vi "Get Class Data.vi"(7 "Object":refnum<class>, 8 "error in (no error)":errorcluster, 10 "Class default data":variant[](array[variant]), 11 "CConfig Variant Accessor in":refnum<class "CConfig Variant Accessor.lvclass">) -> (0 "error out":errorcluster, 2 "Class data":variant[](array[variant]), 3 "CConfig Variant Accessor out":refnum<class "CConfig Variant Accessor.lvclass">, 5 "Object (dup)":refnum<class>)   [LabVIEW 2013, in "CConfig Variant Accessor.lvclass"]
doc: "Copyright 2018, Carya Automatisering, Wiebe Walstra."
uses:
  CConfig Variant Accessor.lvclass
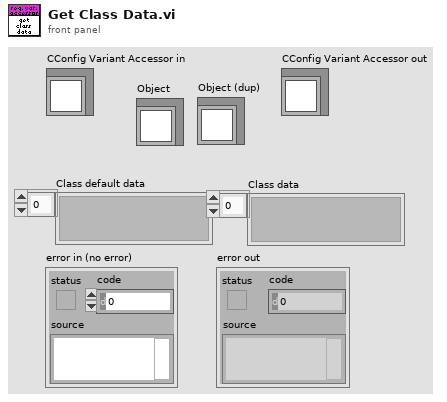
[diagram p1: front panel]
types:
  T1 = cluster{"levels":i32, "h.size":u8, "name size":u8}
  T2 = cluster{"v.major":u16, "v.minor":u16, "v.fix":u16, "v.build":u16}
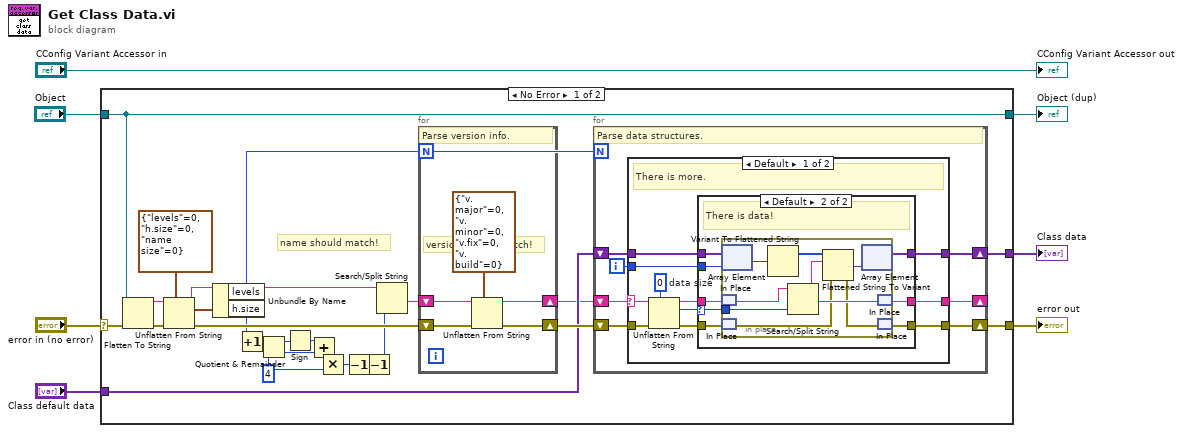
[diagram p0: block diagram]
diagram:
  n1 = case shown="No Error" "error in (no error)" {
    selector: "error in (no error)" -> [w24 w81]
    tunnel: [w23 w81] -> w6
    tunnel: "Object" -> [w22 w80]
    tunnel: [w22 w80] -> w3
    tunnel: "Class default data" -> [w21 w79]
    tunnel: [w20 w79] -> w1
    frame No Error {
      w19 = u8 4 ("y")
      # "name should match!"
      n2 = Flatten To String(anything=w22, error in (no error)=w24) -> (data string=w25:string, error out=w26:errorcluster)  [unwired: 2 in, 1 out]
      n3 = Unflatten From String(type=T1 {"levels"=0, "h.size"=0, "name size"=0}, binary string=w25, error in (no error)=w26) -> (rest of the binary string=w31:string, value=w30:T1, error out=w28:errorcluster)  [unwired: 2 in]
      n4 = Unbundle By Name(w30) -> ("levels"=w29:i32, "h.size"=w11:u8)
      n5 = Increment(x=w11) -> (x+1=w10:u8)
      n6 = Quotient & Remainder(x=w10, y=w19) -> (x-y*floor(x/y)=w16:u8, floor(x/y)=w18:u8)
      n7 = Sign(1:w16) -> (0:w15:u8)
      n8 = Add(x=w15, y=w18) -> (x+y=w17:u8)
      n9 = Multiply(x=w17, y=w19) -> (x*y=w14:u8)
      n10 = Decrement(x=w14) -> (x-1=w9:u8)
      n11 = Decrement(x=w9) -> (x-1=w8:u8)
      n12 = Search/Split String(string=w31, offset (0)=w8) -> (match + rest of string=w12:string)  [unwired: 1 in, 2 out]
      n13 = for {
        N: w29 -> [_]
        shift-right: [w33] -> w27
        shift-left: w28 -> [w36]
        shift-right: [w34] -> w13
        shift-left: w12 -> [w35]
        # "version should match!"
        # "Parse version info."
        n14 = Unflatten From String(type=T2 {"v.major"=0, "v.minor"=0, "v.fix"=0, "v.build"=0}, binary string=w35, error in (no error)=w36) -> (rest of the binary string=w34:string, error out=w33:errorcluster)  [unwired: 2 in, 1 out]
      }
      n15 = for {
        N: w29 -> [_]
        shift-right: [w43] -> w23
        shift-left: w27 -> [w42]
        shift-right: [w44] -> _
        shift-left: w13 -> [w41]
        shift-right: [w39] -> w20
        shift-left: w21 -> [w40]
        i -> [w38]
        # "Parse data structures."
        n16 = case shown="Default" w41 {
          selector: w41 -> [w50 w77]
          tunnel: w42 -> [w55 w78]
          tunnel: [w51 w77] -> w44
          tunnel: [w47 w78] -> w43
          tunnel: w40 -> [w49 w76]
          tunnel: [w48 w76] -> w39
          tunnel: w38 -> [w45 _]
          frame Default {
            w54 = 0  # data size
            # "There is more."
            n17 = Unflatten From String(type=w54, binary string=w50, error in (no error)=w55) -> (rest of the binary string=w52:string, value=w53:i32, error out=w46:errorcluster)  [unwired: 2 in]
            n18 = case shown="Default" w53 {
              selector: w53 -> [_ w66]
              tunnel: w52 -> [w58 w62]
              tunnel: [w58 w61] -> w51
              tunnel: w49 -> [w57 w65]
              tunnel: [w57 w64] -> w48
              tunnel: [w56 w59] -> w47
              tunnel: w46 -> [w56 w60]
              tunnel: w45 -> [_ w63]
              frame 0 {
                # "Data size is 0. Must be default."
              }
              frame Default {
                # "There is data!"
                n19 = in-place {
                  in-place-border: w66 -> [w75]
                  n20 = in-place-array #1(w65, w63) -> (w72:variant)
                  n21 = in-place-match #2(w62) -> (w70:string)
                  n22 = in-place-match #3(w60) -> (w68:errorcluster)
                  n23 = Variant To Flattened String(Variant=w72) -> (1:w73:i16[])  [unwired: 1 out]
                  n24 = Search/Split String(string=w70, offset (0)=w75) -> (substring before match=w74:string, match + rest of string=w69:string)  [unwired: 1 in, 1 out]
                  n25 = Flattened String To Variant(4:w68, 6:w74, 7:w73) -> (0:w67:errorcluster, 3:w71:variant)
                  n26 = in-place-array #1(w71) -> (w64:variant[])  [unwired: 1 out]
                  n27 = in-place-match #2(w69) -> (w61:string)
                  n28 = in-place-match #3(w67) -> (w59:errorcluster)
                }
              }
            }
          }
          frame "" {
            # "No more data, must be default."
          }
        }
      }
    }
    frame Error {
    }
  }
  "error out" <- w6
  "Object (dup)" <- w3
  "Class data" <- w1
  "CConfig Variant Accessor out" <- "CConfig Variant Accessor in"
